vi "Read Config File.vi"(8 "error in (no error)":errorcluster caption="错误输入（无错误）", 11 "TPP demo V2 输入":refnum<class "TPP demo V2.lvclass">) -> (0 "error out":errorcluster caption="错误输出", 3 "TPP demo V2 输出":refnum<class "TPP demo V2.lvclass">)   [LabVIEW 2017, in "TPP demo V2.lvlib" / "TPP demo V2.lvclass"]
uses:
  TPP demo V2.lvclass
  TPP demo V2.lvclass/TPP demo V2.ctl
  <vilib>/Utility/config.llb/Read Key (I32).vi
  <vilib>/Utility/config.llb/NI_LVConfig.lvlib
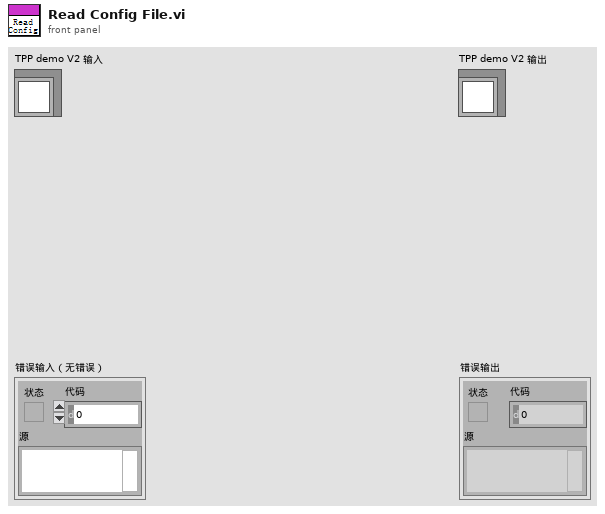
[diagram p1: front panel]
types:
  T1 = typedef "NI_LVConfig.lvlib/Config Data RefNum.ctl" = refnum<k1>
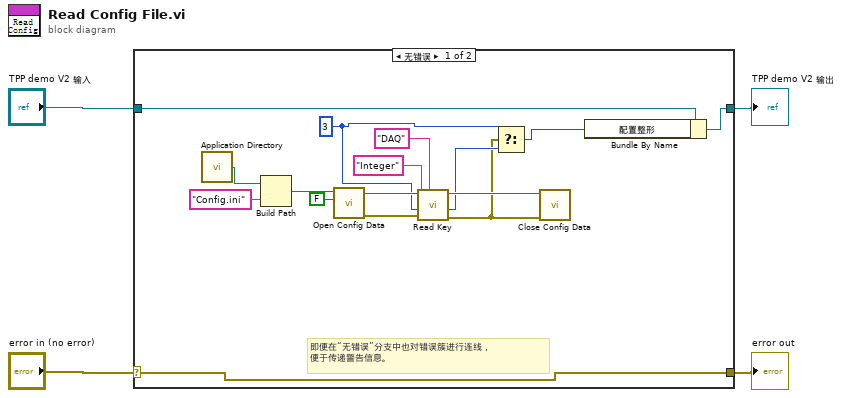
[diagram p0: block diagram]
diagram:
  n1 = case shown="无错误" "error in (no error)" {
    selector: "error in (no error)" -> [w5 w22]
    tunnel: [w5 w22] -> w3
    tunnel: [w11 w21] -> w1
    tunnel: "TPP demo V2 输入" -> [w12 w21]
    frame No Error {
      w7 = 3 ("default value")
      # "即便在“无错误”分支中也对错误簇进行连线，\n便于传递警告信息。"
      n2 = call <vilib>:"Application Directory.vi"() -> ("Application Directory"=w20:path)
      n3 = Build Path(base path=w20, name or relative path="Config.ini" ("名称或相对路径")) -> (appended path=w18:path)
      n4 = call <vilib>:"Open Config Data.vi"("create file if necessary (T)"=FALSE, "configuration file path"=w18) -> ("error out"=w13:errorcluster, "refnum"=w17:T1)  [unwired: 7 in, 1 out]
      n5 = call-poly <vilib>:"Read Key.vi"("section"="DAQ", "error in (no error)"=w13, "default value"=w7, "key"="Integer", "refnum"=w17) -> ("error out"=w8:errorcluster, "value"=w9:i32, "refnum out"=w14:T1)  [unwired: 3 in, 1 out]
      n6 = Select(t=w7, s=w8, f=w9) -> (s? t:f=w6:i32)
      n7 = call <vilib>:"Close Config Data.vi"("error in (no error)"=w8, "refnum"=w14) -> ()  [unwired: 8 in, 2 out]
      n8 = Bundle By Name(cluster=w12, "配置整形"=w6) -> (w11:refnum<class "TPP demo V2.lvclass">)
    }
    frame Error {
    }
  }
  "error out" <- w3
  "TPP demo V2 输出" <- w1
